vi "Write clock id.vi"(8 "error in (no error)":errorcluster, 10 "lv_clockid_t":T1=enum."Monotonic", 11 "Cond in":refnum<class "Cond.lvclass">) -> (0 "error out":errorcluster, 3 "Cond out":refnum<class "Cond.lvclass">)   [LabVIEW 2013, in "Linux RT IPC.lvlib" / "POSIX Threads.lvlib" / "Cond.lvclass"]
uses:
  Cond.lvclass
  <vilib>/NI/NI Linux RT Utilities/Controls/Public/C Enums/clockid_t.ctl
  Cond.lvclass/Cond.ctl
  <vilib>/NI/NI Linux RT Utilities/Linux RT Utilities.lvlib
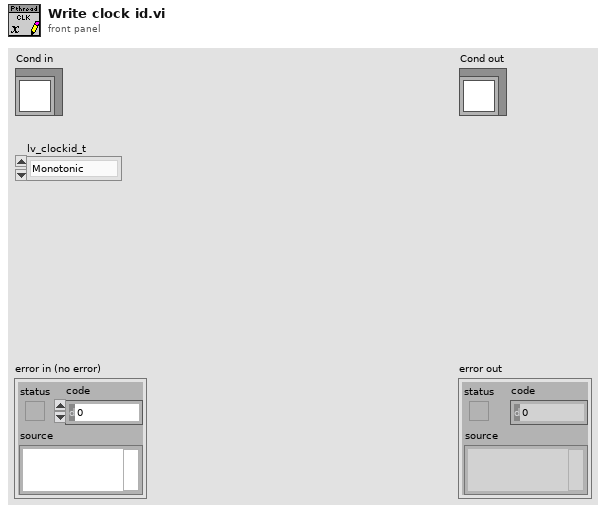
[diagram p1: front panel]
types:
  T1 = typedef "Linux RT Utilities.lvlib/clockid_t.ctl" = enum16{"Realtime", "Monotonic"}
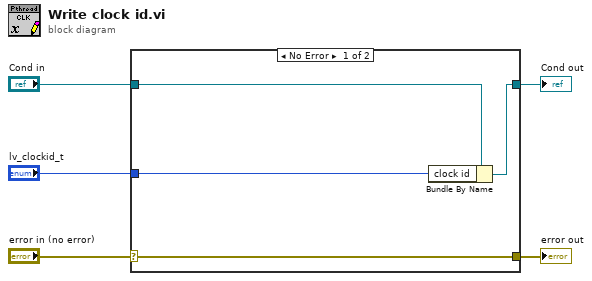
[diagram p0: block diagram]
diagram:
  n1 = case shown="No Error" "error in (no error)" {
    selector: "error in (no error)" -> [w9 w10]
    tunnel: [w9 w10] -> w4
    tunnel: [w7 w11] -> w2
    tunnel: "Cond in" -> [w8 w11]
    tunnel: "lv_clockid_t" -> [w6 _]
    frame No Error {
      n2 = Bundle By Name(cluster=w8, "clock id"=w6) -> (w7:refnum<class "Cond.lvclass">)
    }
    frame Error {
    }
  }
  "error out" <- w4
  "Cond out" <- w2
